vi "response.vi"(7 "result (0)":i32, 8 "error in (no error)":errorcluster, 10 "ID":i32) -> (0 "error out":errorcluster, 2 "reply":string)   [LabVIEW 2020]
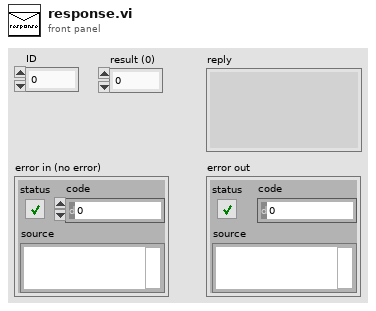
[diagram p1: front panel]
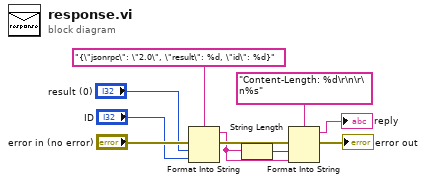
[diagram p0: block diagram]
diagram:
  n1 = Format Into String(format string="{\"jsonrpc\": \"2.0\", \"result\": %d, \"id\": %d}", error in="error in (no error)", "result (0)", "ID") -> (resulting string=w4:string, error out=w8:errorcluster)  [unwired: 1 in]
  n2 = String Length(string=w4) -> (length=w5:i32)
  n3 = Format Into String(format string="Content-Length: %d\r\n\r\n%s", error in=w8, w5, w4) -> (resulting string=→"reply":string, error out=→"error out":errorcluster)  [unwired: 1 in]
